vi "Signal Comparison_.vi"() -> ()   [LabVIEW 2010]
uses:
  <vilib>/Analysis/NI_AALBase.lvlib
panel:
  out "sum":dbl
  out "Waveform Graph 2":dbl[](graph)
  out "error 2":i32
  out "error":i32
  out "Waveform Graph":dbl[](graph)
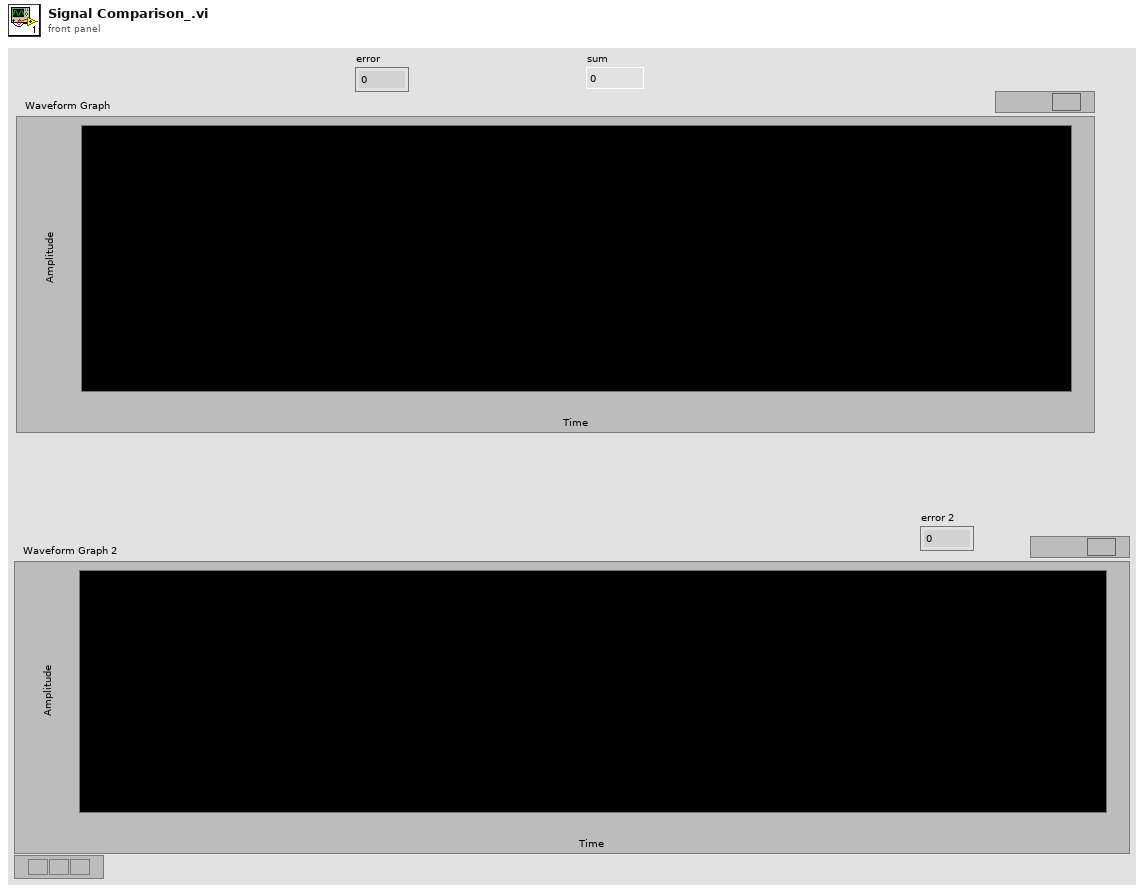
[diagram p1: front panel]
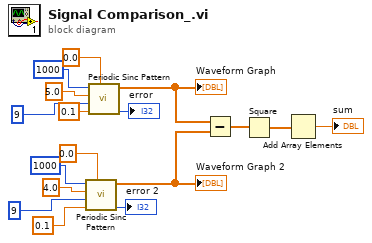
[diagram p0: block diagram]
diagram:
  n1 = call <vilib>:"Periodic Sinc Pattern.vi"("delay (s)"=0.0, "delta t (s)"=0.1, "order"=9, "amplitude"=4.0, "samples"=1000) -> ("error"=→"error 2":i32, "Periodic Sinc Pattern"=w4:dbl[])  [unwired: 5 in]
  "Waveform Graph 2" <- w4
  n2 = call <vilib>:"Periodic Sinc Pattern.vi"("delay (s)"=0.0, "delta t (s)"=0.1, "order"=9, "amplitude"=5.0, "samples"=1000) -> ("error"=→"error":i32, "Periodic Sinc Pattern"=w5:dbl[])  [unwired: 5 in]
  "Waveform Graph" <- w5
  n3 = Subtract(x=w5, y=w4) -> (x-y=w3:dbl[])
  n4 = Square(x=w3) -> (x^2=w2:dbl[])
  n5 = Add Array Elements(numeric array=w2) -> (sum=→"sum":dbl)
